vi "FixedQueryTicklish.vi"(8 "byte count":u32, 9 "write buffer":string, 11 "Serial USB port name":refnum<visa-resource-name>) -> (0 "error out":errorcluster, 1 "Result string":string, 3 "Serial USB port name out":refnum<visa-resource-name>)   [LabVIEW 2015]
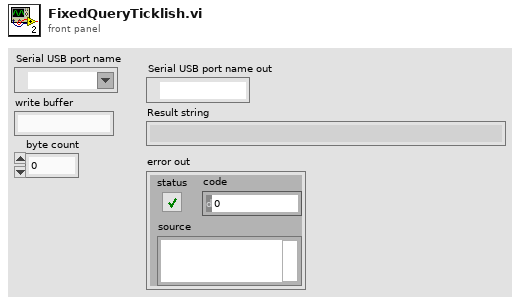
[diagram p1: front panel]
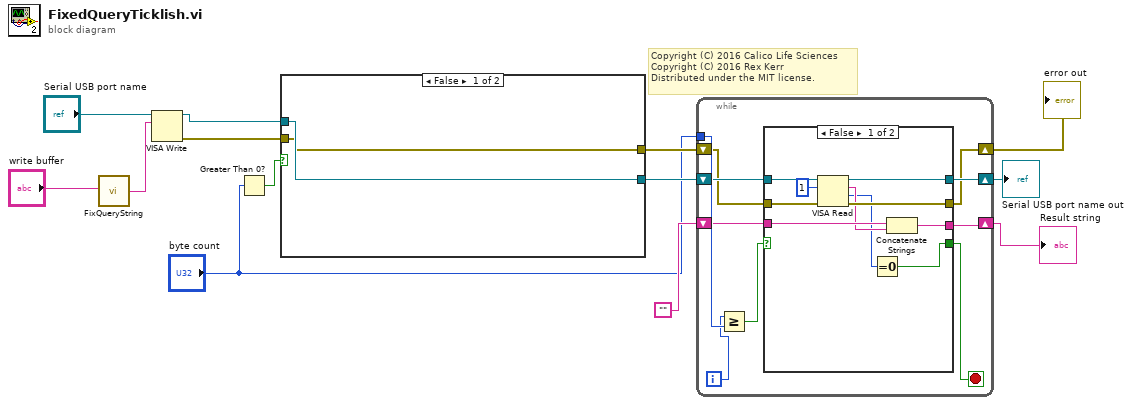
[diagram p0: block diagram]
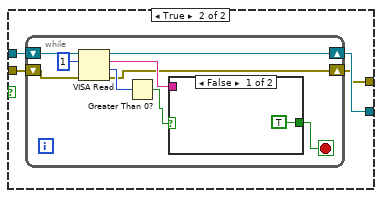
[diagram p2: hidden frame]
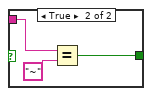
[diagram p3: hidden frame]
diagram:
  # "Copyright (C) 2016 Calico Life Sciences\nCopyright (C) 2016 Rex Kerr\nDistributed under the MIT license."
  n1 = call "FixQueryString.vi"("write buffer"="write buffer") -> ("write buffer fixed"=w1:string)  [unwired: 4 in]
  n2 = VISA Write(VISA resource name="Serial USB port name", write buffer=w1) -> (VISA resource name out=w12:refnum<visa-resource-name>, error out=w11:errorcluster)  [unwired: 1 in, 1 out]
  n3 = Greater Than 0?(x="byte count") -> (x > 0?=w3:bool)
  n4 = case shown="False" w3 {
    tunnel: w12 -> [w15 w19]
    tunnel: w11 -> [w14 w18]
    tunnel: [w15 w17] -> w10
    tunnel: [w14 w16] -> w9
    frame False {
    }
    frame True {
      n5 = while {
        shift-right: [w27] -> w17
        shift-left: w19 -> [w28]
        shift-right: [w21] -> w16
        shift-left: w18 -> [w22]
        stop <- w23 stop-if-true
        n6 = VISA Read(VISA resource name=w28, byte count=u32 1, error in (no error)=w22) -> (VISA resource name out=w27:refnum<visa-resource-name>, read buffer=w24:string, return count=w25:u32, error out=w21:errorcluster)
        n7 = Greater Than 0?(x=w25) -> (x > 0?=w20:bool)
        n8 = case shown="False" w20 {
          tunnel: w24 -> [_ w32]
          tunnel: [TRUE w30] -> w23
          frame False {
          }
          frame True {
            n9 = Equal?(x=w32, y="~") -> (x = y?=w30:bool)
          }
        }
      }
    }
  }
  n10 = while {
    tunnel: "byte count" -> [w42]
    shift-right: [w37] -> w7
    shift-left: w10 -> [w38]
    shift-right: [w35] -> w5
    shift-left: w9 -> [w36]
    shift-right: [w33] -> w6
    shift-left: "" -> [w34]
    i -> [w41]
    stop <- w39 stop-if-true
    n11 = Greater Or Equal?(x=w41, y=w42) -> (x >= y?=w40:bool)
    n12 = case shown="False" w40 {
      selector: w40 -> [_ w56]
      tunnel: [w44 w56] -> w39
      tunnel: w38 -> [w52 w55]
      tunnel: [w51 w55] -> w37
      tunnel: w36 -> [w49 w54]
      tunnel: [w48 w54] -> w35
      tunnel: w34 -> [w47 w53]
      tunnel: [w43 w53] -> w33
      frame False {
        n13 = VISA Read(VISA resource name=w52, byte count=u32 1, error in (no error)=w49) -> (VISA resource name out=w51:refnum<visa-resource-name>, read buffer=w46:string, return count=w45:u32, error out=w48:errorcluster)
        n14 = Equal To 0?(x=w45) -> (x = 0?=w44:bool)
        n15 = Concatenate Strings(w47, w46) -> (w43:string)
      }
      frame True {
      }
    }
  }
  "Serial USB port name out" <- w7
  "Result string" <- w6
  "error out" <- w5
